vi "Calculate Setpoint.vi"(8 "error in (no error)":errorcluster, 10 "time (sec)":dbl, 11 "Sawtooth in":refnum<class "Sawtooth.lvclass">) -> (0 "error out":errorcluster, 1 "type":string, 2 "setpoint":dbl, 3 "Sawtooth out":refnum<class "Sawtooth.lvclass">, 5 "testing?":bool)   [LabVIEW 2020, in "Sawtooth.lvclass"]
uses:
  Sawtooth.lvclass
  C:/Users/jharw/Documents/1 Folder to Rule them All/UMD/Inflation-Apparatus/src/Inflation Test/Parameter Class/IA Test Parameters.lvclass
  Sawtooth.lvclass/Sawtooth.ctl
  IA Test Parameters.lvclass/IA Test Parameters.ctl
  IA Test Parameters.lvclass
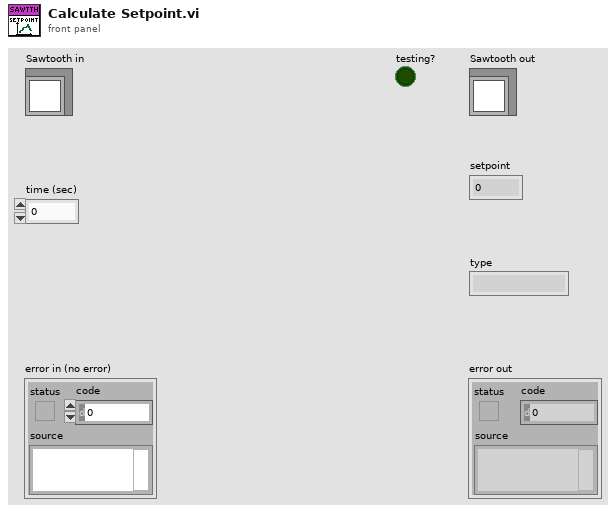
[diagram p1: front panel]
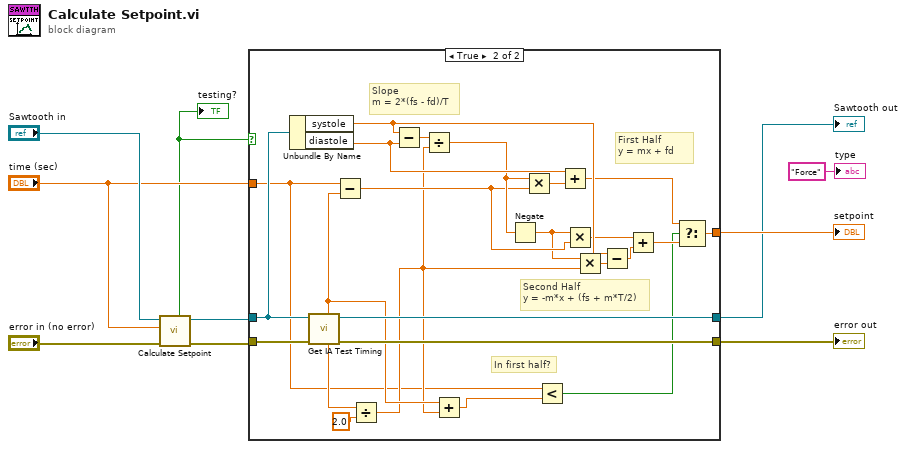
[diagram p0: block diagram]
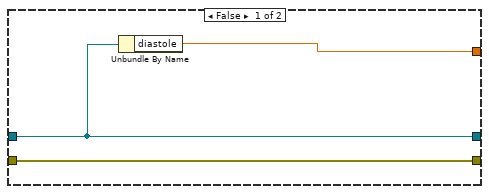
[diagram p2: hidden frame]
diagram:
  n1 = call-parent "Calculate Setpoint.vi"("error in (no error)"="error in (no error)", "time (sec)"="time (sec)", "IA Test Parameters in"="Sawtooth in") -> ("error out"=w8:errorcluster, "IA Test Parameters out"=w7:refnum<class "Sawtooth.lvclass">, "testing?"=w5:bool)  [unwired: 4 in, 2 out]
  "testing?" <- w5
  n2 = case shown="True" w5 {
    tunnel: w7 -> [w12 w36]
    tunnel: "time (sec)" -> [_ w14]
    tunnel: [w13 w24] -> w3
    tunnel: w8 -> [w11 w35]
    tunnel: [w11 w34] -> w4
    tunnel: [w12 w33] -> w1
    frame False {
      n3 = Unbundle By Name(w12) -> ("diastole"=w13:dbl)
    }
    frame True {
      # "Second Half\ny = -m*x + (fs + m*T/2)"
      # "In first half?"
      # "First Half\ny = mx + fd"
      # "Slope\nm = 2*(fs - fd)/T"
      n4 = Unbundle By Name(w36) -> ("systole"=w25:dbl, "diastole"=w29:dbl)
      n5 = call "Get IA Test Timing.vi"("error in (no error)"=w35, "IA Test Parameters in"=w36) -> ("error out"=w34:errorcluster, "IA Test Parameters out"=w33:refnum<class "Sawtooth.lvclass">, "test period (sec)"=w32:dbl, "time delay (sec)"=w30:dbl)  [unwired: 4 in, 2 out]
      n6 = Subtract(x=w14, y=w30) -> (x-y=w26:dbl)
      n7 = Divide(x=w32, y=2.0) -> (x/y=w16:dbl)
      n8 = Subtract(x=w25, y=w29) -> (x-y=w37:dbl)
      n9 = Divide(x=w37, y=w16) -> (x/y=w27:dbl)
      n10 = Add(x=w30, y=w16) -> (x+y=w15:dbl)
      n11 = Negate(x=w27) -> (-x=w18:dbl)
      n12 = Multiply(x=w27, y=w26) -> (x*y=w28:dbl)
      n13 = Less?(x=w14, y=w15) -> (x < y?=w21:bool)
      n14 = Add(x=w29, y=w28) -> (x+y=w22:dbl)
      n15 = Multiply(x=w18, y=w26) -> (x*y=w20:dbl)
      n16 = Multiply(x=w18, y=w16) -> (x*y=w19:dbl)
      n17 = Subtract(x=w25, y=w19) -> (x-y=w17:dbl)
      n18 = Add(x=w20, y=w17) -> (x+y=w23:dbl)
      n19 = Select(t=w22, s=w21, f=w23) -> (s? t:f=w24:dbl)
    }
  }
  "error out" <- w4
  "Sawtooth out" <- w1
  "setpoint" <- w3
  "type" <- "Force" ("type")
